vi "GVZeitenZyklen.vi"() -> ()   [LabVIEW 2017]
panel:
  out "ZyklusNummernGesamt":i32[](array[numeric])
  out "ZyklusNummern":i32[](array[numeric])
  out "Big Ben, Methodenzeit, Zykluszeit0, Zykluszeit1, Zykluszeit2A, Zykluszeit2B":dbl[](array[numeric])
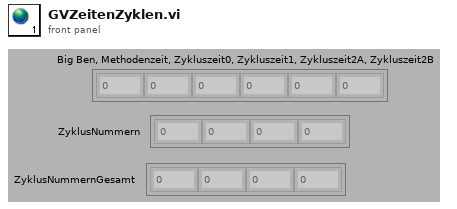
[diagram p1: front panel]
diagram:
